vi "Update Drawing When Mouse Up.vi"(8 "error in (no error)":errorcluster, 10 "Graphic":refnum<class "Graphic.lvclass">, 11 "Canvas in":refnum<class "Canvas.lvclass">) -> (0 "error out":errorcluster, 3 "Canvas out":refnum<class "Canvas.lvclass">)   [LabVIEW 2015, in "Canvas.lvclass"]
uses:
  Canvas.lvclass
  Graphic/Graphic.lvclass
  Canvas.lvclass/Canvas.ctl
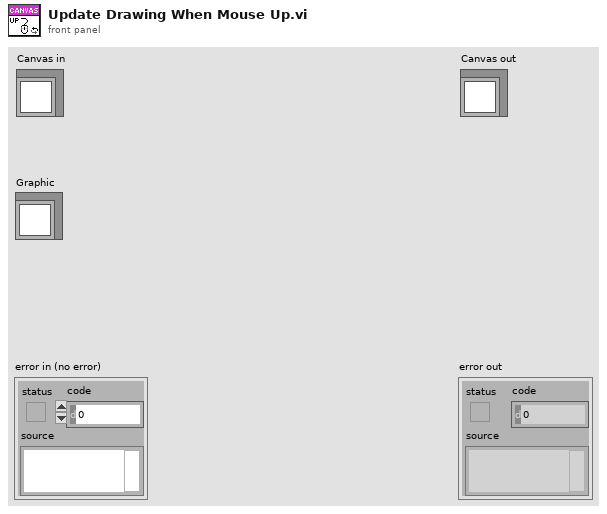
[diagram p1: front panel]
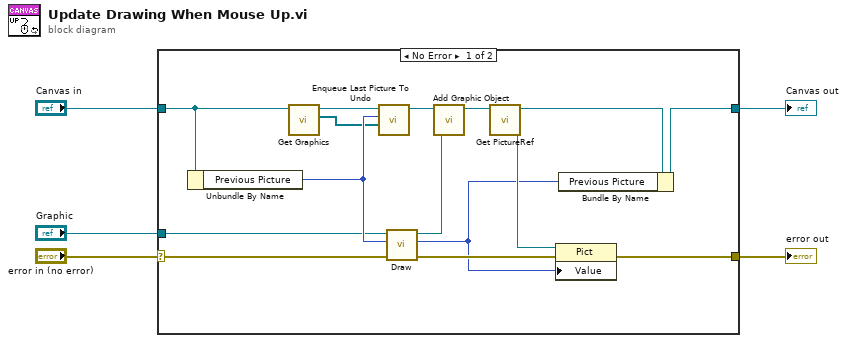
[diagram p0: block diagram]
diagram:
  n1 = case shown="No Error" "error in (no error)" {
    selector: "error in (no error)" -> [w16 w22]
    tunnel: [w15 w22] -> w4
    tunnel: [w20 w21] -> w2
    tunnel: "Canvas in" -> [w19 w21]
    tunnel: "Graphic" -> [w17 _]
    frame No Error {
      n2 = Unbundle By Name(w19) -> ("Previous Picture"=w18:picture)
      n3 = call "Get Graphics.vi"("Canvas in"=w19) -> ("Graphics"=w9:refnum<class "Graphic.lvclass">[], "Canvas out"=w10:refnum<class "Canvas.lvclass">)  [unwired: 8 in, 1 out]
      n4 = call "Enqueue Last Picture To Undo.vi"("Graphics"=w9, "Last Picture"=w18, "Canvas in"=w10) -> ("Canvas out"=w8:refnum<class "Canvas.lvclass">)  [unwired: 7 in, 1 out]
      n5 = call-dynamic "Draw.vi"("error in (no error)"=w16, "Picture in"=w18, "Graphic in"=w17) -> ("error out"=w14:errorcluster, "Picture out"=w11:picture, "Graphic out"=w12:refnum<class "Graphic.lvclass">)  [unwired: 6 in]
      n6 = call "Add Graphic Object.vi"("Graphic"=w12, "Canvas in"=w8) -> ("Canvas out"=w7:refnum<class "Canvas.lvclass">)  [unwired: 7 in, 2 out]
      n7 = call "Get PictureRef.vi"("Canvas in"=w7) -> ("PictureRef"=w13:refnum<vi>, "Canvas out"=w6:refnum<class "Canvas.lvclass">)  [unwired: 8 in, 1 out]
      n8 = property class="Pict"(reference=w13, error in=w14, "Value"=w11) -> (error out=w15:errorcluster)  [unwired: 1 out]
      n9 = Bundle By Name(cluster=w6, "Previous Picture"=w11) -> (w20:refnum<class "Canvas.lvclass">)
    }
    frame Error {
    }
  }
  "error out" <- w4
  "Canvas out" <- w2
